vi "Configure Percentage.vi"(8 "error in (no error)":errorcluster, 9 "Reference (0)":dbl, 10 "Enable Percentage Measurement (F: Disable)":bool, 11 "VISA resource name":refnum<visa-resource-name>) -> (0 "error out":errorcluster, 3 "VISA resource name out":refnum<visa-resource-name>)   [LabVIEW 2021, in "GWInstek  GDM8351.lvlib"]
doc: "Configures the percentage measurement.\n\nRuns the following equation:\n\n((ReadingX - Reference) / Reference) x 100%"
uses:
  <instrlib>/GWInstek  GDM8351/GWInstek  GDM8351.lvlib
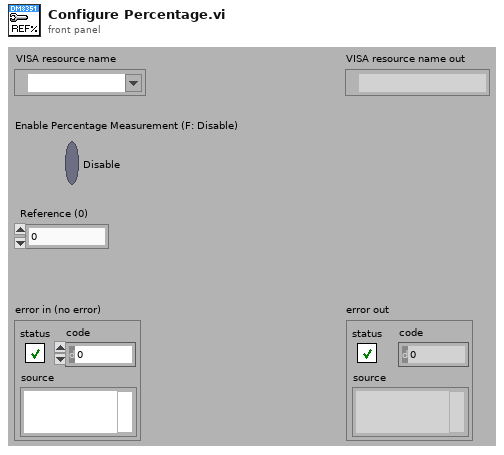
[diagram p1: front panel]
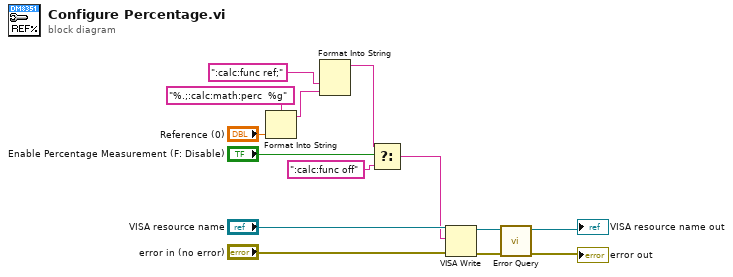
[diagram p0: block diagram]
diagram:
  n1 = Format Into String(format string="%.;:calc:math:perc  %g", "Reference (0)") -> (resulting string=w2:string)  [unwired: 2 in, 1 out]
  n2 = Format Into String(":calc:func ref;", w2) -> (resulting string=w4:string)  [unwired: 3 in, 1 out]
  n3 = Select(t=w4, s="Enable Percentage Measurement (F: Disable)", f=":calc:func off") -> (s? t:f=w3:string)
  n4 = VISA Write(VISA resource name="VISA resource name", write buffer=w3, error in (no error)="error in (no error)") -> (VISA resource name out=w14:refnum<visa-resource-name>, error out=w13:errorcluster)  [unwired: 1 out]
  n5 = call <instrlib>:"Error Query.vi"("error in (no error)"=w13, "VISA resource name"=w14) -> ("error out"=→"error out":errorcluster, "VISA resource name out"=→"VISA resource name out":refnum<visa-resource-name>)  [unwired: 6 in, 2 out]
